vi "Write RegistryKey.vi"(8 "error in (no error)":errorcluster, 10 "RegistryKey":string, 11 "Attribute.Identity in":refnum<class "Attribute.Identity.lvclass">) -> (0 "error out":errorcluster, 3 "Attribute.Identity out":refnum<class "Attribute.Identity.lvclass">)   [LabVIEW 2013, in "Attribute.Identity.lvclass"]
uses:
  Attribute.Identity.lvclass
  Attribute.Identity.lvclass/Attribute.Identity.ctl
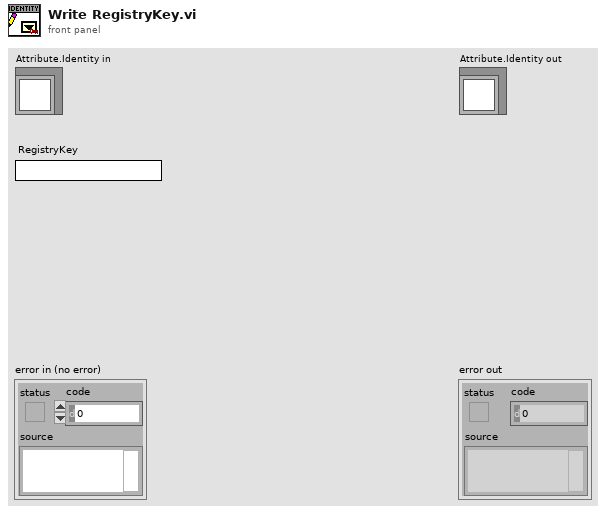
[diagram p1: front panel]
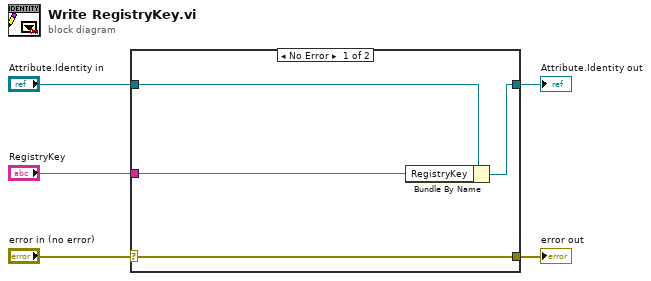
[diagram p0: block diagram]
diagram:
  n1 = case shown="No Error" "error in (no error)" {
    selector: "error in (no error)" -> [w9 w10]
    tunnel: [w9 w10] -> w4
    tunnel: [w7 w11] -> w2
    tunnel: "Attribute.Identity in" -> [w8 w11]
    tunnel: "RegistryKey" -> [w6 _]
    frame No Error {
      n2 = Bundle By Name(cluster=w8, "RegistryKey"=w6) -> (w7:refnum<class "Attribute.Identity.lvclass">)
    }
    frame Error {
    }
  }
  "error out" <- w4
  "Attribute.Identity out" <- w2
